vi "ENA_setMarker.vi"(5 "Step_Freq(GHz)":dbl=0.5 format="%#_13g", 7 "Start_Freq(GHz)":dbl=26.5 format="%#_13g", 8 "error in":errorcluster, 9 "Simulation":bool, 10 "Markers_num":i32=11, 11 "VISA IN":refnum<visa-resource-name>="TCPIP0::192.168.100.12::inst0::INSTR") -> (0 "error out":errorcluster, 3 "Marker_array":dbl[](array[numeric]))   [LabVIEW 2023, in "Keysight.lvlib"]
uses:
  Keysight.lvlib
  CTL/Keysight_VNA.ctl
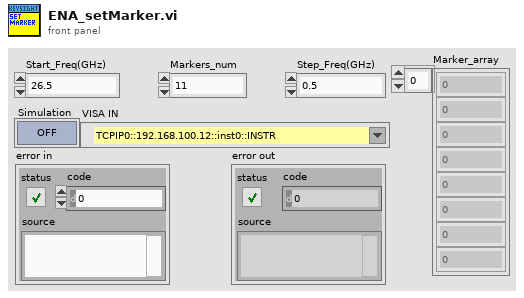
[diagram p1: front panel]
types:
  T1 = typedef "Keysight_VNA.ctl" = enum16{"Init", "queryMarker", "setSweepPoint", "setMarkerFreq", "setMeasureFormat", "setFreqStartStop", "setMarkerOnOFF", "setMarkerFormat_LOGP", "setMeasPAR_S", "setTriggerSingle", "Trigger_Save_SnP", "Trigger_Single", "Close"}
  T2 = cluster{"setSweepPoint":i32, "Meas":i32, "Mark":i32, "Freq_GHz":dbl, "Start_Freq(GHz)":dbl, "Stop_Freq(GHz)":dbl, "sParameter":i32}
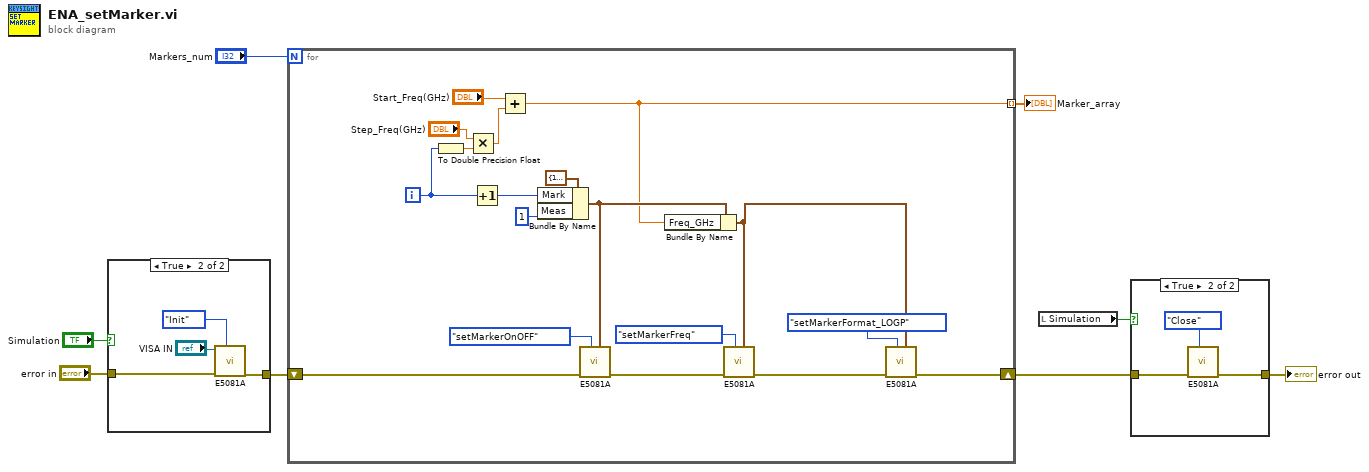
[diagram p0: block diagram]
diagram:
  n1 = case shown="True" "Simulation" {
    tunnel: "error in" -> [w9 w13]
    tunnel: [w9 w10] -> w7
    frame False {
    }
    frame True {
      n2 = call "E5081A.vi"("Function_VNA"=Keysight_VNA."Init", "error in"=w13, "VISA IN"="VISA IN") -> ("error out"=w10:errorcluster)  [unwired: 7 in, 1 out]
    }
  }
  n3 = for {
    N: "Markers_num" -> [_]
    shift-right: [w17] -> w6
    shift-left: w7 -> [w31]
    tunnel: [w14] -> w1 mode=indexing
    i -> [w26]
    n4 = To Double Precision Float(number=w26) -> (double precision float=w24:dbl)
    n5 = Multiply(x="Step_Freq(GHz)", y=w24) -> (x*y=w22:dbl)
    n6 = Increment(x=w26) -> (x+1=w19:i32)
    n7 = Add(x="Start_Freq(GHz)", y=w22) -> (x+y=w14:dbl)
    n8 = Bundle By Name(cluster=T2 {"setSweepPoint"=11, "Meas"=1, "Mark"=0, "Freq_GHz"=0.0, "Start_Freq(GHz)"=0.0, "Stop_Freq(GHz)"=0.0, "sParameter"=1} ("Input"), "Mark"=w19, "Meas"=1) -> (w21:T2)
    n9 = call "E5081A.vi"("Input"=w21, "Function_VNA"=Keysight_VNA."setMarkerOnOFF", "error in"=w31) -> ("error out"=w28:errorcluster)  [unwired: 7 in, 1 out]
    n10 = Bundle By Name(cluster=w21, "Freq_GHz"=w14) -> (w15:T2)
    n11 = call "E5081A.vi"("Input"=w15, "Function_VNA"=Keysight_VNA."setMarkerFreq", "error in"=w28) -> ("error out"=w18:errorcluster)  [unwired: 7 in, 1 out]
    n12 = call "E5081A.vi"("Input"=w15, "Function_VNA"=Keysight_VNA."setMarkerFormat_LOGP", "error in"=w18) -> ("error out"=w17:errorcluster)  [unwired: 7 in, 1 out]
  }
  "Marker_array" <- w1
  n13 = local read "Simulation"() -> (w2:bool)
  n14 = case shown="True" w2 {
    tunnel: w6 -> [w32 w35]
    tunnel: [w32 w33] -> w4
    frame False {
    }
    frame True {
      n15 = call "E5081A.vi"("Function_VNA"=Keysight_VNA."Close", "error in"=w35) -> ("error out"=w33:errorcluster)  [unwired: 8 in, 1 out]
    }
  }
  "error out" <- w4
